vi "Drive_Tag.vi"(0 "Timeout (ms)":dbl, 1 "Acceptable Error":dbl, 2 "Red/Blue":bool, 3 "Botpose Target":dbl) -> ()   [LabVIEW 2020]
uses:
  Robot Global Data.vi
  <vilib>/Rock Robotics/WPI/RobotDrive/WPI_RobotDriveArcadeDrive_Standard(NoSaturation).vi
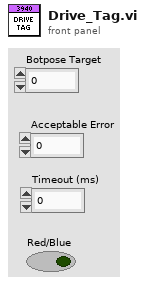
[diagram p1: front panel]
types:
  T1 = typedef "WPI_RobotDriveDevRef.ctl" = cluster{"DevStatus":errorcluster, "Motors[]":T2[], "Square Inputs":bool, "Max Output":dbl}
  T2 = typedef "WPI_MotorControlDeviceRef.ctl" = cluster{"DeviceStatus":errorcluster, "Type":T3, "PWM":cluster{"PWM Channel":T4, "DeadBand":T5}, "CAN":cluster{"Device Number":u8, "SetOutput VI Ref":variant, "GetOutput VI Ref":variant, "Enable VI Ref":variant, "Disable VI Ref":variant, "Data":variant}, "Invert":bool, "DIO PWM":cluster{"PWM \"Enable\" Channel":T4, "DIOChannel":T6, "PWM Rate":dbl}}
  T3 = typedef "WPI_MotorControlType.ctl" = enum16{"PWM", "CAN", "DIO PWM"}
  T4 = typedef "FPGA_DIOPWMChannel.ctl" = enum8{"PWM 0", "PWM 1", "PWM 2", "PWM 3", "PWM 4", "PWM 5", "PWM 6", "PWM 7", "PWM 8", "PWM 9", "PWM MXP 0", "PWM MXP 1", "PWM MXP 2", "PWM MXP 3", "PWM MXP 4", "PWM MXP 5", "PWM MXP 6", "PWM MXP 7", "PWM MXP 8", "PWM MXP 9", "Invalid"}
  T5 = typedef "WPI_PWMDeadband.ctl" = cluster{"Name":string, "maxPositivePwm":i32, "minPositivePwm":i32, "centerPwm":i32, "maxNegativePwm":i32, "minNegativePwm":i32, "angularRange":u16}
  T6 = typedef "FPGA_DIOChannel.ctl" = enum8{"DIO 0", "DIO 1", "DIO 2", "DIO 3", "DIO 4", "DIO 5", "DIO 6", "DIO 7", "DIO 8", "DIO 9", "DIO MXP 0", "DIO MXP 1", "DIO MXP 2", "DIO MXP 3", "DIO MXP 4", "DIO MXP 5", "DIO MXP 6", "DIO MXP 7", "DIO MXP 8", "DIO MXP 9", "DIO MXP 10", "DIO MXP 11", "DIO MXP 12", "DIO MXP 13", "DIO MXP 14", "DIO MXP 15", "SPI Port CS1", "SPI Port CS2", "SPI Port CS3", "SPI Port MISO", "SPI Port MOSI", "Invalid"}
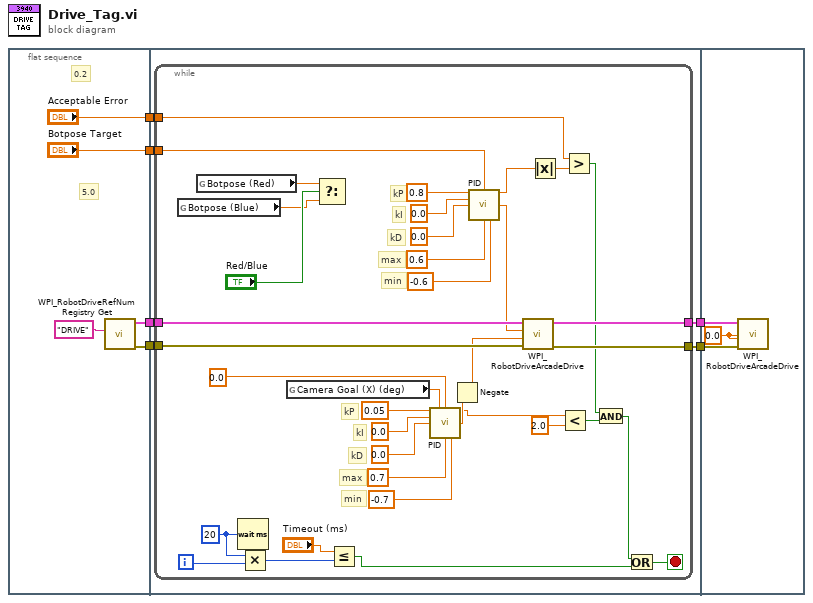
[diagram p0: block diagram]
diagram:
  n1 = flat-sequence {
    tunnel: [w10] -> w6
    tunnel: [w9] -> w5
    tunnel: ["Botpose Target"] -> w4
    tunnel: ["Acceptable Error"] -> w3
    tunnel: w6 -> [w16]
    tunnel: w5 -> [w15]
    tunnel: w4 -> [w17]
    tunnel: w3 -> [w14]
    tunnel: [w13] -> w2
    tunnel: [w12] -> w1
    tunnel: w2 -> [w57]
    tunnel: w1 -> [w56]
    frame #0 {
      # "0.2"
      # "5.0"
      n2 = call <vilib>:"WPI_RobotDriveRefNum Registry Get.vi"("refnum name"="DRIVE") -> ("error out"=w9:errorcluster, "RobotDriveDevRef"=w10:T1)  [unwired: 9 in]
    }
    frame #1 {
      n3 = while {
        tunnel: w17 -> [w54]
        tunnel: w16 -> [w48]
        tunnel: w15 -> [w47]
        tunnel: w14 -> [w38]
        tunnel: [w31] -> w13
        tunnel: [w30] -> w12
        i -> [w34]
        stop <- w33 stop-if-true
        w35 = u32 20 ("milliseconds to wait")
        # "min"
        # "max"
        # "kD"
        # "kI"
        # "kP"
        # "min"
        # "max"
        # "kD"
        # "kI"
        # "kP"
        n4 = global read "Robot Global Data.vi" "Botpose (Blue)"() -> (w18:dbl)
        n5 = global read "Robot Global Data.vi" "Botpose (Red)"() -> (w20:dbl)
        n6 = Wait (ms)(milliseconds to wait=w35) -> ()  [unwired: 1 out]
        n7 = Multiply(x=w35, y=w34) -> (x*y=w36:u32)
        n8 = global read "Robot Global Data.vi" "Camera Goal (X) (deg)"() -> (w46:dbl)
        n9 = Select(t=w20, s="Red/Blue", f=w18) -> ()  [unwired: 1 out]
        n10 = Less Or Equal?(x="Timeout (ms)", y=w36) -> (x <= y?=w32:bool)
        n11 = call "PID.vi"("Kp"=0.05, "Process Variable"=w46, "Goal"=0.0, "Ki"=0.0, "Kd"=0.0, "Max Ouput"=0.7, "Min Output"=-0.7) -> ("Current Error"=w24:dbl, "Command"=w29:dbl)  [unwired: 6 in, 1 out]
        n12 = Negate(x=w29) -> (-x=w27:dbl)
        n13 = call "PID.vi"("Kp"=0.8, "Goal"=w54, "Ki"=0.0, "Kd"=0.0, "Max Ouput"=0.6, "Min Output"=-0.6) -> ("Current Error"=w40:dbl, "Command"=w28:dbl)  [unwired: 7 in, 1 out]
        n14 = call-poly <vilib>:"WPI_RobotDriveArcadeDrive.vi"("error in (no error)"=w47, "Y axis value"=w27, "X axis value"=w28, "RobotDriveDevRef"=w48) -> ("error out"=w30:errorcluster, "RobotDriveDevRef"=w31:T1)  [unwired: 5 in, 1 out]
        n15 = Absolute Value(x=w40) -> (abs(x)=w39:dbl)
        n16 = Less?(x=w24, y=2.0) -> (x < y?=w25:bool)
        n17 = Greater?(x=w38, y=w39) -> (0:w26:bool)
        n18 = And(x=w26, y=w25) -> (x .and. y?=w22:bool)
        n19 = Or(x=w22, y=w32) -> (x .or. y?=w33:bool)
      }
    }
    frame #2 {
      w55 = 0.0 ("X axis value")
      n20 = call-poly <vilib>:"WPI_RobotDriveArcadeDrive.vi"("error in (no error)"=w56, "Y axis value"=w55, "X axis value"=w55, "RobotDriveDevRef"=w57) -> ()  [unwired: 5 in, 3 out]
    }
  }
